vi "Measurement Logic.vi"(8 "error in":errorcluster, 11 "Measurement Configuration":T3={"Input Voltage in V"=4.0, "Nominal Output Voltage in V"=3.3, "Start"=0.03, "Stop"=0.43, "Step"=0.01, "Input SMU"="DPS_4145_1/1", "Load SMU"="DPS_4145_1/3", "Input DMM"="DMM1", "Load DMM"="DMM2"}) -> (0 "error out":errorcluster, 3 "Measurement Results":T2 {"Load Regulation (mV/mA)" format="%#.5g"})   [LabVIEW 2020, in "LoadRegulation.lvlib"]
uses:
  LoadRegulation.lvlib
  Measurement Configuration.ctl
  Measurement Results.ctl
  Reusables/TestResults.ctl
  Reusables/TestInputs.ctl
  Reusables/Advanced Settings.ctl
  Reusables/Prepare Fn Configurations.ctl
  Reusables/Load Output Function.ctl
  Reusables/Stimulus And Measure.ctl
  1892a527-43d9-4058-946b-211879b654a6.vi
panel:
  out "Load Regulation (mV/mA)":dbl format="%#.3g"
  out "Load Regulation (%)":dbl format="%#.3g"
  out "Test Results":T1
  out "Load Regulation":cluster{"Iload (mA)":dbl[], "Vout (V)":dbl[]}(graph)
  # "Below outputs could be used to debug or verify when we run this vi as standalone"
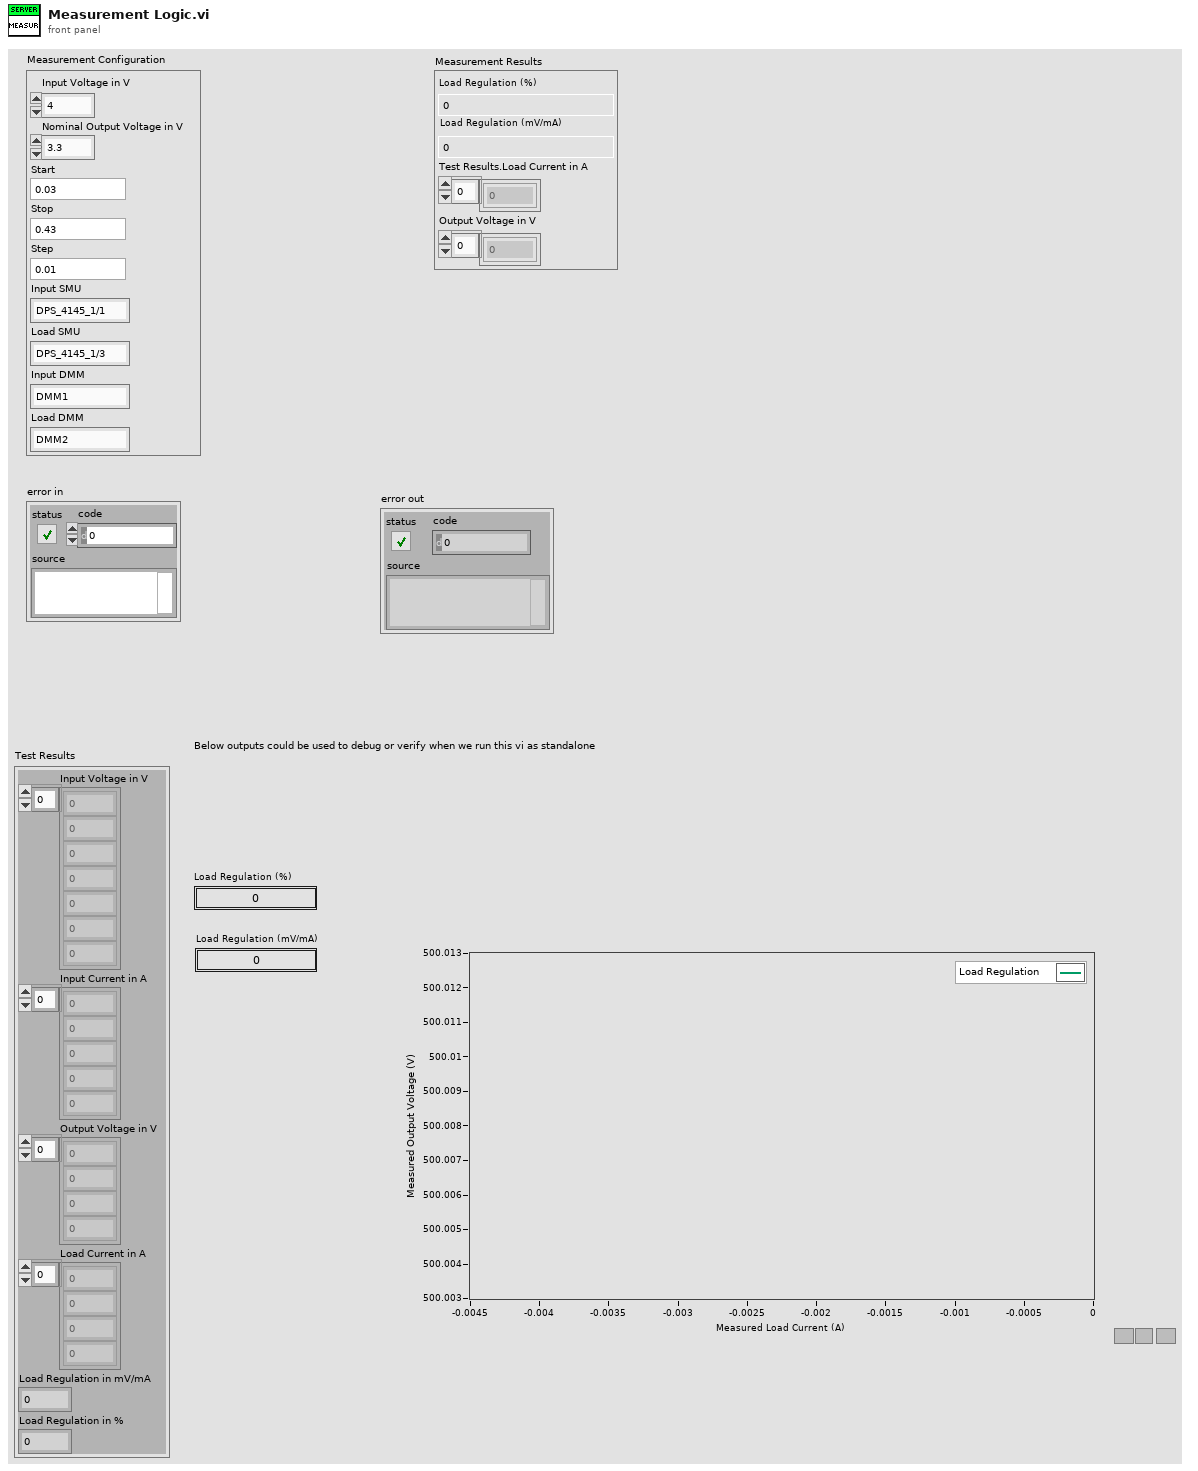
[diagram p1: front panel]
types:
  T1 = typedef "LoadRegulation.lvlib/TestResults.ctl" = cluster{"Input Voltage in V":dbl[], "Input Current in A":dbl[], "Output Voltage in V":dbl[], "Load Current in A":dbl[], "Load Regulation in mV/mA":dbl, "Load Regulation in %":dbl}
  T2 = typedef "LoadRegulation.lvlib/Measurement Results.ctl" = cluster{"Load Regulation (%)":dbl, "Load Regulation (mV/mA)":dbl, "Test Results.Load Current in A":dbl[], "Output Voltage in V":dbl[]}
  T3 = typedef "LoadRegulation.lvlib/Measurement Configuration.ctl" = cluster{"Input Voltage in V":dbl, "Nominal Output Voltage in V":dbl, "Start":dbl, "Stop":dbl, "Step":dbl, "Input SMU":string, "Load SMU":string, "Input DMM":string, "Load DMM":string}
  T4 = typedef "LoadRegulation.lvlib/TestInputs.ctl" = cluster{"Input Voltage in V":dbl, "Load Current in A":dbl[], "Nominal Output Voltage in V":dbl, "Advance Setting":T5}
  T5 = typedef "Advanced Settings.ctl" = cluster{"Prepare":T6, "Stimulus And Measure":T8}
  T6 = typedef "Prepare Fn Configurations.ctl" = cluster{"Load SMU Output Function":T7}
  T7 = typedef "Load Output Function.ctl" = enum16{"VoltageSource", "CurrentSource"}
  T8 = typedef "Stimulus And Measure.ctl" = cluster{"Loop Delay in milliSecond":u32}
  T9 = cluster{"Test Inputs":T4, "Test Results":T1, "Test Results[][]":string[][], "Input SMU":refnum<k15>, "Input DMM":refnum<k15>, "Load DMM":refnum<k15>, "Load SMU":refnum<k15>}
  T10 = cluster{"Load Current in A":dbl[], "Output Voltage in V":dbl[]}
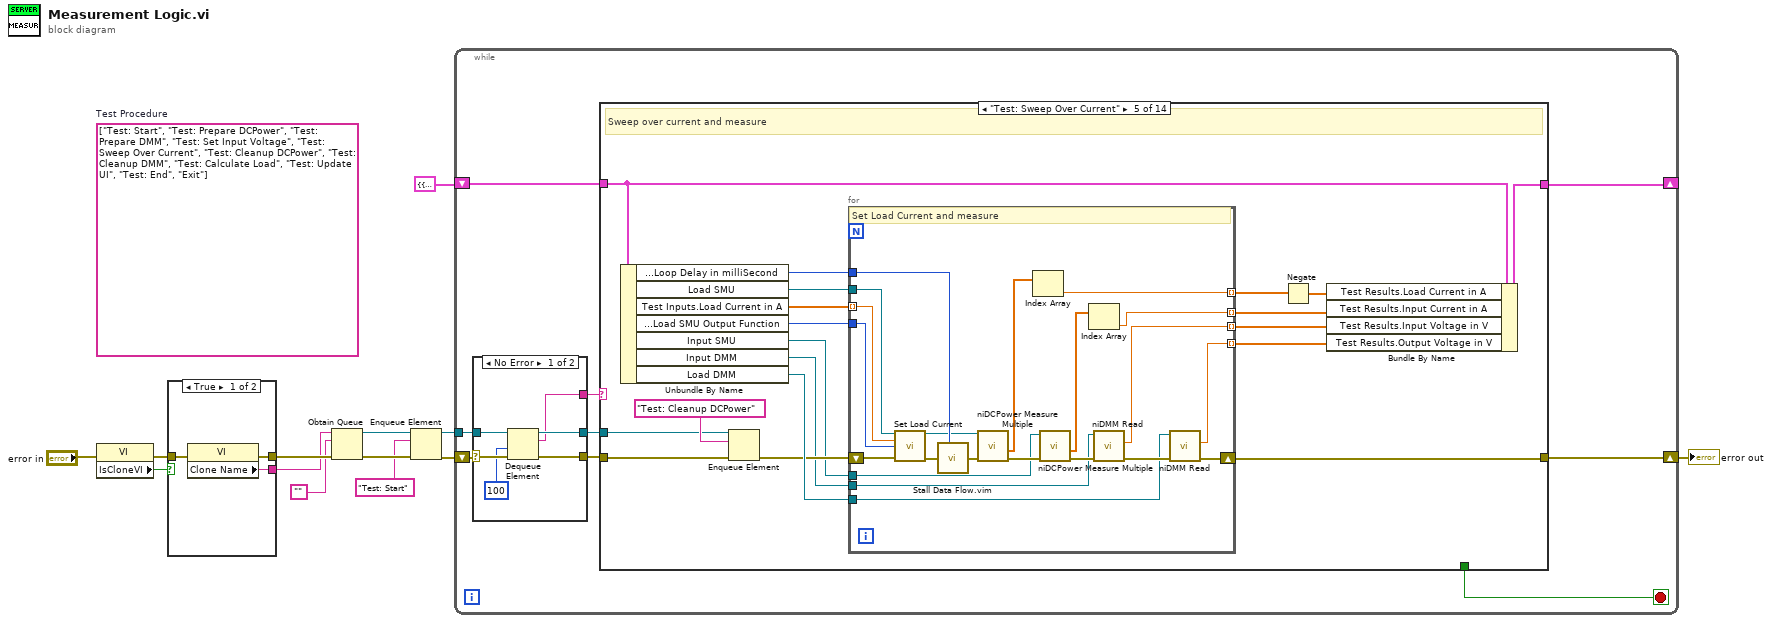
[diagram p0: block diagram]
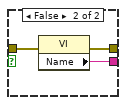
[diagram p2: hidden frame]
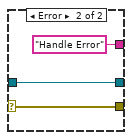
[diagram p3: hidden frame]
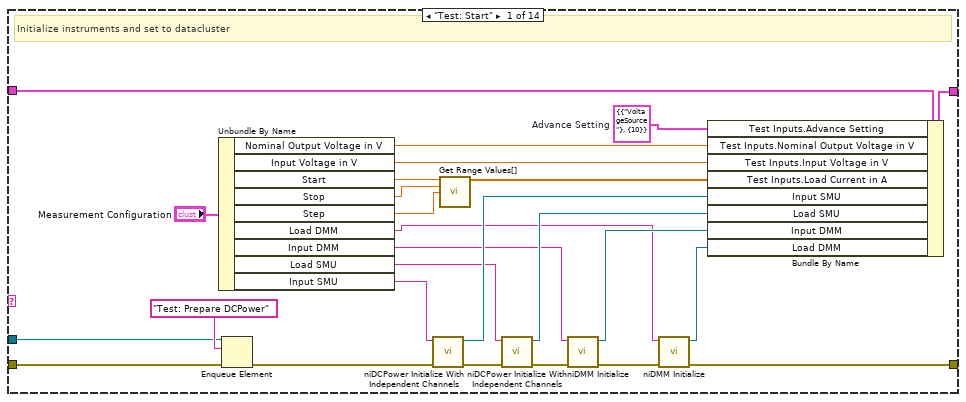
[diagram p4: hidden frame]
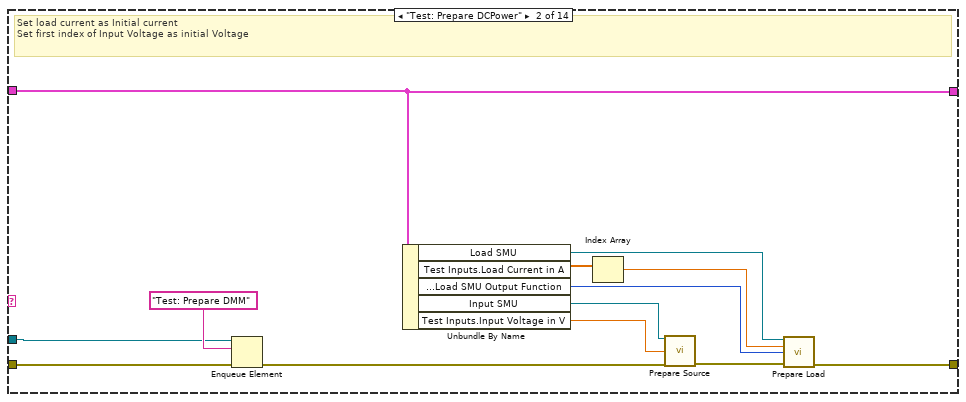
[diagram p5: hidden frame]
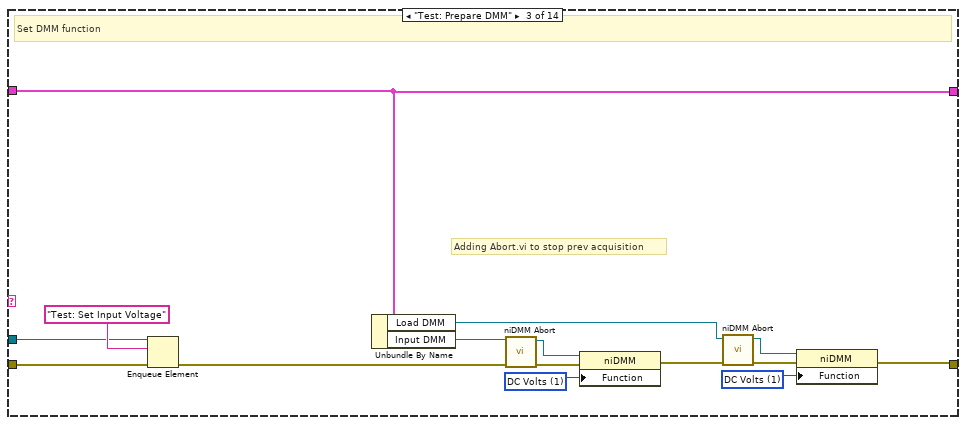
[diagram p6: hidden frame]
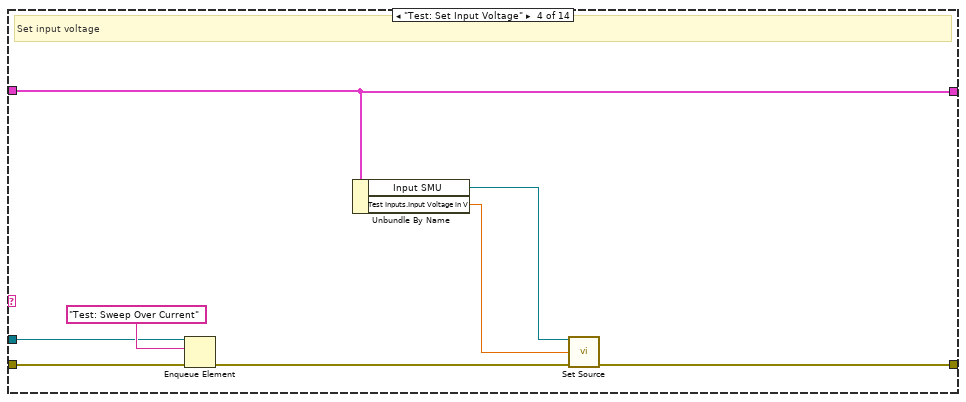
[diagram p7: hidden frame]
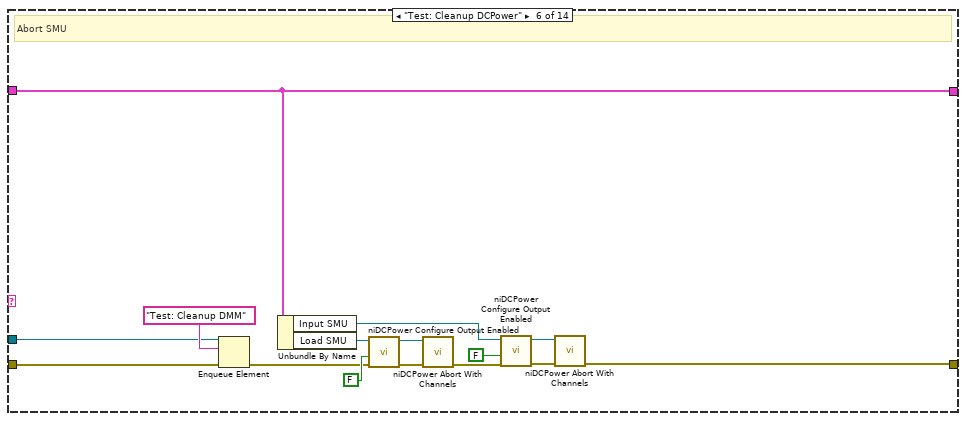
[diagram p8: hidden frame]
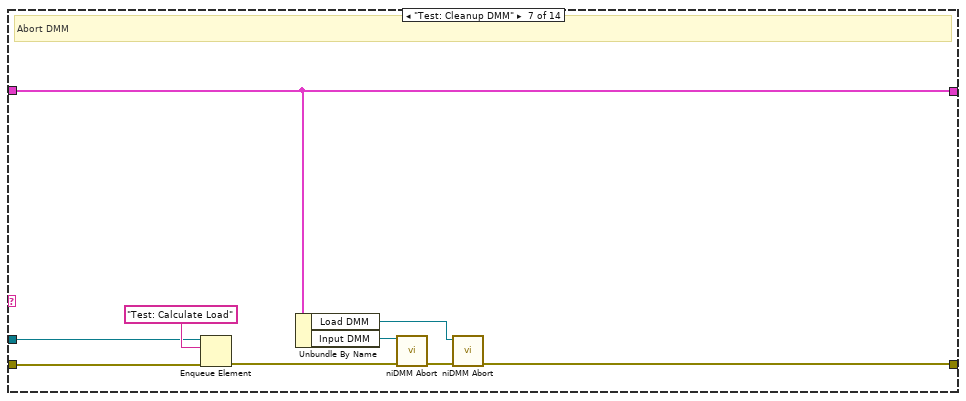
[diagram p9: hidden frame]
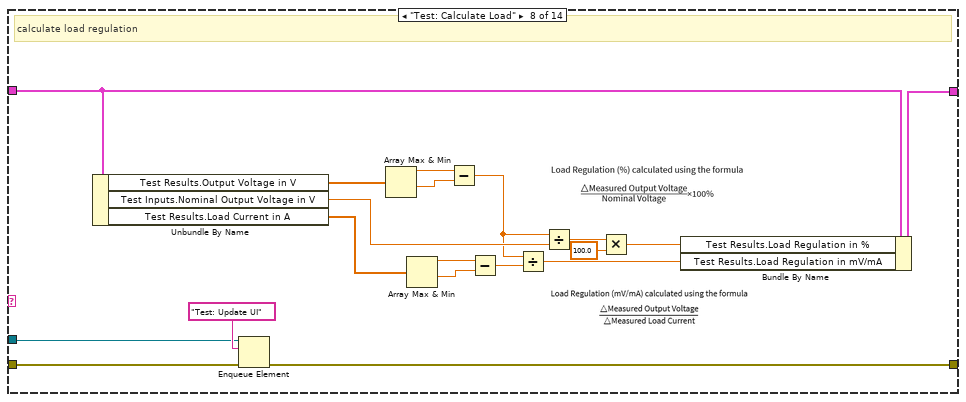
[diagram p10: hidden frame]
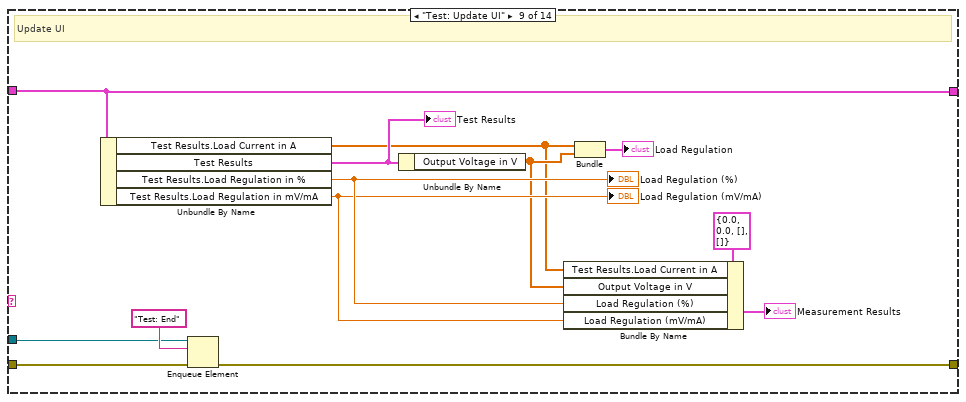
[diagram p11: hidden frame]
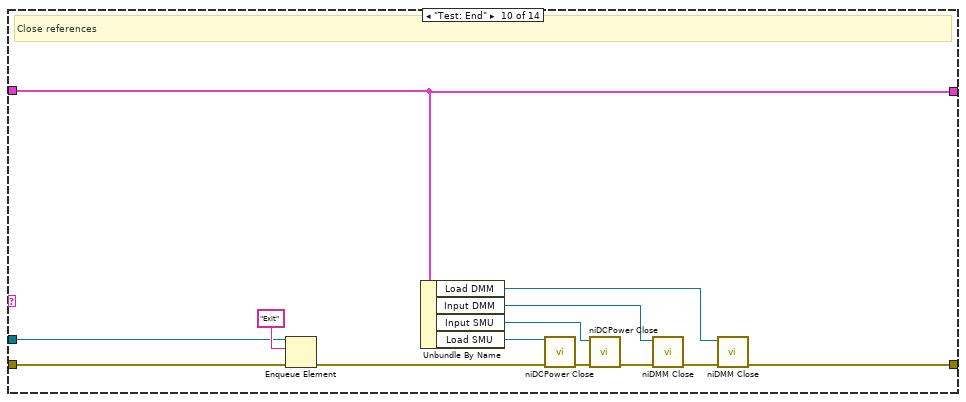
[diagram p12: hidden frame]
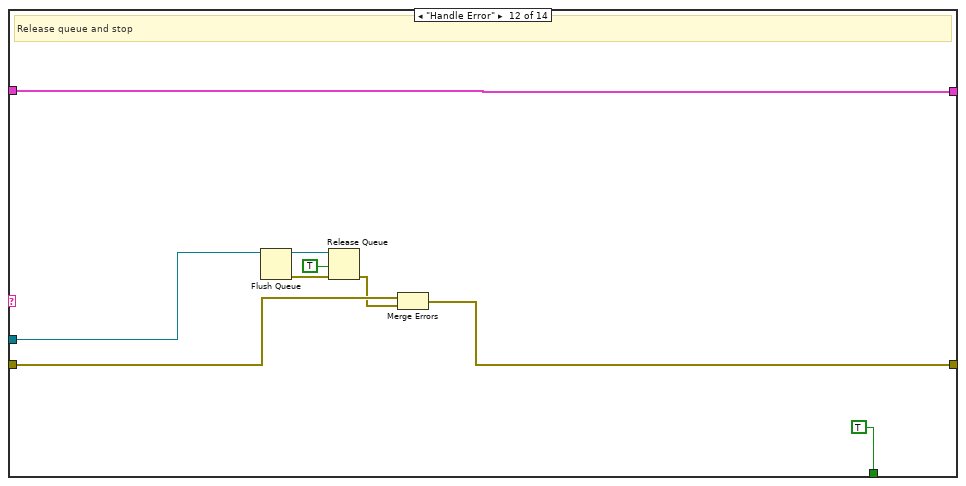
[diagram p14: hidden frame]
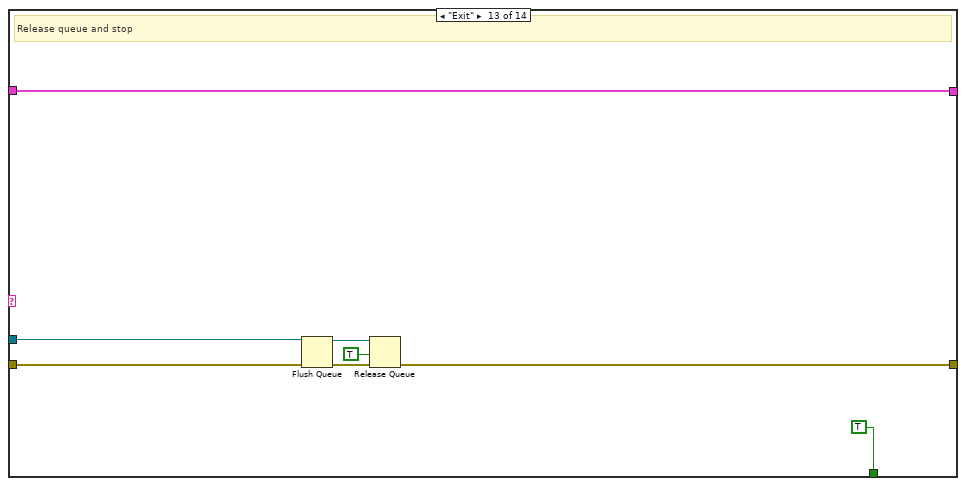
[diagram p15: hidden frame]
diagram:
  (unwired) string[] ["Test: Start", "Test: Prepare DCPower", "Test: Prepare DMM", "Test: Set Input Voltage", "Test: Sweep Over Current", "Test: Cleanup DCPower", "Test: Cleanup DMM", "Test: Calculate Load", "Test: Update UI", "Test: End", "Exit"]  # Test Procedure
  n1 = property class="VI"(error in="error in") -> (error out=w4:errorcluster, "IsCloneVI"=w5:bool)  [unwired: 1 in, 1 out]
  n2 = case shown="True" w5 {
    tunnel: [w16 w19] -> w11
    tunnel: [w15 w18] -> w10
    tunnel: w4 -> [w14 w17]
    frame True {
      n3 = property class="VI"(error in=w14) -> (error out=w16:errorcluster, "Clone Name"=w15:string)  [unwired: 1 in, 1 out]
    }
    frame False {
      n4 = property class="VI"(error in=w17) -> (error out=w19:errorcluster, "Name"=w18:string)  [unwired: 1 in, 1 out]
    }
  }
  n5 = Obtain Queue(name (unnamed)=w10, element data type="", error in (no error)=w11) -> (queue out=w8:refnum<queue>, error out=w9:errorcluster)  [unwired: 2 in, 1 out]
  n6 = Enqueue Element(queue=w8, element="Test: Start", error in (no error)=w9) -> (queue out=w2:refnum<queue>, error out=w1:errorcluster)  [unwired: 1 in, 1 out]
  n7 = while {
    tunnel: w2 -> [w23]
    shift-right: [w28] -> w12
    shift-left: w1 -> [w24]
    shift-right: [w26] -> _
    shift-left: T9 {"Test Inputs"={"Input Voltage in V"=0.0, "Load Current in A"=[], "Nominal Output Voltage in V"=0.0, "Advance Setting"={"Prepare"={"Load SMU Output Function"=enum."VoltageSource"}, "Stimulus And Measure"={"Loop Delay in milliSecond"=1}}}, "Test Results"={"Input Voltage in V"=[], "Input Current in A"=[], "Output Voltage in V"=[], "Load Current in A"=[], "Load Regulation in mV/mA"=0.0, "Load Regulation in %"=0.0}, "Test Results[][]"=[], "Input SMU"="", "Input DMM"="", "Load DMM"="", "Load SMU"=""} -> [w27]
    stop <- w25 stop-if-true
    n8 = case shown="No Error" w24 {
      selector: w24 -> [w34 w37]
      tunnel: [w33 w37] -> w20
      tunnel: w23 -> [w32 w36]
      tunnel: [w31 w36] -> w21
      tunnel: [w30 "Handle Error"] -> w22
      frame No Error {
        n9 = Dequeue Element(queue=w32, timeout in ms (-1)=100, error in (no error)=w34) -> (queue out=w31:refnum<queue>, element=w30:string, error out=w33:errorcluster)  [unwired: 1 out]
      }
      frame Error {
      }
    }
    n10 = case shown="\"Test: Sweep Over Current\"" w22 {
      tunnel: w21 -> [w43 w66 w79 w94 w106 w140 w155 w164 w183 w196 _ w211 w220 _]
      tunnel: w20 -> [w42 w67 w77 w92 w104 w142 w156 w165 w184 w197 w210 w217 w222 w228]
      tunnel: [w58 w70 w82 w96 w110 w151 w161 w166 w185 w202 w210 w218 w221 w228] -> w28
      tunnel: w27 -> [w62 w75 w88 w99 w108 w150 w163 w168 w193 w208 w209 w219 w227 w229]
      tunnel: [w63 w75 w88 w99 w109 w150 w163 w169 w193 w208 w209 w219 w227 w229] -> w26
      tunnel: [_ _ _ _ _ _ _ _ _ _ _ TRUE TRUE _] -> w25
      frame "Test: Start" {
        w40 = T5 {"Prepare"={"Load SMU Output Function"=enum."VoltageSource"}, "Stimulus And Measure"={"Loop Delay in milliSecond"=10}}  # Advance Setting
        # "Initialize instruments and set to datacluster"
        n11 = Unbundle By Name("Measurement Configuration") -> ("Nominal Output Voltage in V"=w53:dbl, "Input Voltage in V"=w38:dbl, "Start"=w51:dbl, "Stop"=w50:dbl, "Step"=w49:dbl, "Load DMM"=w45:string, "Input DMM"=w46:string, "Load SMU"=w47:string, "Input SMU"=w48:string)
        n12 = Enqueue Element(queue=w43, element="Test: Prepare DCPower", error in (no error)=w42) -> (error out=w41:errorcluster)  [unwired: 1 in, 2 out]
        n13 = call <instrlib>:"niDCPower Initialize With Independent Channels.vi"("error in (no error)"=w41, "resource name"=w48) -> ("error out"=w57:errorcluster, "instrument handle out"=w61:refnum<k15>)  [unwired: 8 in]
        n14 = call "Get Range Values[].vi"("Start"=w51, "Stop"=w50, "Step Size"=w49) -> ("Values[]"=w39:dbl[])  [unwired: 12 in]
        n15 = call <instrlib>:"niDCPower Initialize With Independent Channels.vi"("error in (no error)"=w57, "resource name"=w47) -> ("error out"=w56:errorcluster, "instrument handle out"=w54:refnum<k15>)  [unwired: 8 in]
        n16 = call <instrlib>:"niDMM Initialize.vi"("error in (no error)"=w56, "Instrument Descriptor"=w46) -> ("error out"=w59:errorcluster, "instrument handle out"=w55:refnum<k15>)  [unwired: 8 in]
        n17 = call <instrlib>:"niDMM Initialize.vi"("error in (no error)"=w59, "Instrument Descriptor"=w45) -> ("error out"=w58:errorcluster, "instrument handle out"=w60:refnum<k15>)  [unwired: 8 in]
        n18 = Bundle By Name(cluster=w62, "Test Inputs.Advance Setting"=w40, "Test Inputs.Nominal Output Voltage in V"=w53, "Test Inputs.Input Voltage in V"=w38, "Test Inputs.Load Current in A"=w39, "Input SMU"=w61, "Load SMU"=w54, "Input DMM"=w55, "Load DMM"=w60) -> (w63:T9)
      }
      frame "Test: Prepare DCPower" {
        # "Set load current as Initial current\nSet first index of Input Voltage as initial Voltage"
        n19 = Enqueue Element(queue=w66, element="Test: Prepare DMM", error in (no error)=w67) -> (error out=w68:errorcluster)  [unwired: 1 in, 2 out]
        n20 = Unbundle By Name(w75) -> ("Load SMU"=w73:refnum<k15>, "Test Inputs.Load Current in A"=w72:dbl[], "Test Inputs.Advance Setting.Prepare.Load SMU Output Function"=w64:T7, "Input SMU"=w74:refnum<k15>, "Test Inputs.Input Voltage in V"=w76:dbl)
        n21 = Index Array(array=w72) -> (element=w65:dbl)  [unwired: 1 in]
        n22 = call "Prepare Source.vi"("instrument handle"=w74, "Initial Voltage Level (V)"=w76, "error in (no error)"=w68) -> ("error out"=w71:errorcluster)  [unwired: 12 in]
        n23 = call "Prepare Load.vi"("instrument handle"=w73, "Load Current Level (A)"=w65, "Load Output Function"=w64, "error in (no error)"=w71) -> ("error out"=w70:errorcluster)  [unwired: 11 in]
      }
      frame "Test: Prepare DMM" {
        w84 = 1 items=["DC Volts"=1, "AC Volts"=2, "DC Current"=3, "AC Current"=4, "2-Wire Resistance"=5, "4-Wire Resistance"=101, "Frequency"=104, "Period"=105, "AC Volts DC Coupled"=1001, "Diode"=1002, "Waveform Voltage"=1003, "Waveform Current"=1004, "Capacitance"=1005, "Inductance"=1006, "Temperature"=108] ("Configuration:Function")
        w91 = 1 items=["DC Volts"=1, "AC Volts"=2, "DC Current"=3, "AC Current"=4, "2-Wire Resistance"=5, "4-Wire Resistance"=101, "Frequency"=104, "Period"=105, "AC Volts DC Coupled"=1001, "Diode"=1002, "Waveform Voltage"=1003, "Waveform Current"=1004, "Capacitance"=1005, "Inductance"=1006, "Temperature"=108] ("Configuration:Function")
        # "Adding Abort.vi to stop prev acquisition"
        # "Set DMM function"
        n24 = Enqueue Element(queue=w79, element="Test: Set Input Voltage", error in (no error)=w77) -> (error out=w78:errorcluster)  [unwired: 1 in, 2 out]
        n25 = Unbundle By Name(w88) -> ("Load DMM"=w81:refnum<k15>, "Input DMM"=w87:refnum<k15>)
        n26 = call <instrlib>:"niDMM Abort.vi"("error in (no error)"=w78, "instrument handle"=w87) -> ("error out"=w90:errorcluster, "instrument handle out"=w89:refnum<k15>)  [unwired: 8 in]
        n27 = property class="niDMM"(reference=w89, error in=w90, "Function"=w91) -> (error out=w83:errorcluster)  [unwired: 1 out]
        n28 = call <instrlib>:"niDMM Abort.vi"("error in (no error)"=w83, "instrument handle"=w81) -> ("error out"=w85:errorcluster, "instrument handle out"=w86:refnum<k15>)  [unwired: 8 in]
        n29 = property class="niDMM"(reference=w86, error in=w85, "Function"=w84) -> (error out=w82:errorcluster)  [unwired: 1 out]
      }
      frame "Test: Set Input Voltage" {
        # "Set input voltage"
        n30 = Enqueue Element(queue=w94, element="Test: Sweep Over Current", error in (no error)=w92) -> (error out=w93:errorcluster)  [unwired: 1 in, 2 out]
        n31 = Unbundle By Name(w99) -> ("Input SMU"=w98:refnum<k15>, "Test Inputs.Input Voltage in V"=w97:dbl)
        n32 = call "Set Source.vi"("instrument handle in"=w98, "Vin in V"=w97, "error in (no error)"=w93) -> ("error out"=w96:errorcluster)  [unwired: 11 in, 1 out]
      }
      frame "Test: Sweep Over Current" {
        # "Sweep over current and measure"
        n33 = Unbundle By Name(w108) -> ("Test Inputs.Advance Setting.Stimulus And Measure.Loop Delay in milliSecond"=w116:u32, "Load SMU"=w118:refnum<k15>, "Test Inputs.Load Current in A"=w117:dbl[], "Test Inputs.Advance Setting.Prepare.Load SMU Output Function"=w103:T7, "Input SMU"=w100:refnum<k15>, "Input DMM"=w101:refnum<k15>, "Load DMM"=w115:refnum<k15>)
        n34 = Enqueue Element(queue=w106, element="Test: Cleanup DCPower", error in (no error)=w104) -> (error out=w105:errorcluster)  [unwired: 1 in, 2 out]
        n35 = for {
          tunnel: w118 -> [w138]
          tunnel: w117 -> [w121] mode=indexing
          tunnel: w116 -> [w136]
          tunnel: w101 -> [w129]
          tunnel: w115 -> [w128]
          tunnel: [w122] -> w114 mode=indexing
          tunnel: [w123] -> w113 mode=indexing
          tunnel: [w127] -> w112 mode=indexing
          tunnel: [w126] -> w111 mode=indexing
          shift-right: [w125] -> w110
          shift-left: w105 -> [w139]
          tunnel: w103 -> [w120]
          tunnel: w100 -> [w119]
          # "Set Load Current and measure"
          n36 = call "Set Load Current.vi"("instrument handle in"=w138, "current level"=w121, "OutputFunction"=w120, "error in (no error)"=w139) -> ("instrument handle out"=w124:refnum<k15>, "error out"=w137:errorcluster)  [unwired: 10 in]
          n37 = call "Stall Data Flow.vim"("value in"=w137, "milliseconds to wait"=w136) -> ("value out"=w130:errorcluster)  [unwired: 1 out]
          n38 = call <instrlib>:"niDCPower Measure Multiple.vi"("error in (no error)"=w130, "instrument handle"=w124) -> ("error out"=w132:errorcluster, "current measurements"=w135:dbl[])  [unwired: 6 in, 2 out]
          n39 = Index Array(array=w135) -> (element=w123:dbl)  [unwired: 1 in]
          n40 = call <instrlib>:"niDCPower Measure Multiple.vi"("error in (no error)"=w132, "instrument handle"=w119) -> ("error out"=w131:errorcluster, "current measurements"=w133:dbl[])  [unwired: 6 in, 2 out]
          n41 = Index Array(array=w133) -> (element=w122:dbl)  [unwired: 1 in]
          n42 = call <instrlib>:"niDMM Read.vi"("error in (no error)"=w131, "instrument handle"=w129) -> ("error out"=w134:errorcluster, "Measurement"=w127:dbl)  [unwired: 7 in, 1 out]
          n43 = call <instrlib>:"niDMM Read.vi"("error in (no error)"=w134, "instrument handle"=w128) -> ("error out"=w125:errorcluster, "Measurement"=w126:dbl)  [unwired: 7 in, 1 out]
        }
        n44 = Negate(x=w113) -> (-x=w102:dbl[])
        n45 = Bundle By Name(cluster=w108, "Test Results.Load Current in A"=w102, "Test Results.Input Current in A"=w114, "Test Results.Input Voltage in V"=w112, "Test Results.Output Voltage in V"=w111) -> (w109:T9)
      }
      frame "Test: Cleanup DCPower" {
        # "Abort SMU"
        n46 = Enqueue Element(queue=w140, element="Test: Cleanup DMM", error in (no error)=w142) -> (error out=w141:errorcluster)  [unwired: 1 in, 2 out]
        n47 = Unbundle By Name(w150) -> ("Input SMU"=w149:refnum<k15>, "Load SMU"=w144:refnum<k15>)
        n48 = call <instrlib>:"niDCPower Configure Output Enabled.vi"("error in (no error)"=w141, "output enabled"=FALSE, "instrument handle"=w144) -> ("error out"=w145:errorcluster, "instrument handle out"=w148:refnum<k15>)  [unwired: 7 in]
        n49 = call <instrlib>:"niDCPower Abort With Channels.vi"("error in (no error)"=w145, "instrument handle"=w148) -> ("error out"=w146:errorcluster)  [unwired: 8 in, 1 out]
        n50 = call <instrlib>:"niDCPower Configure Output Enabled.vi"("error in (no error)"=w146, "output enabled"=FALSE, "instrument handle"=w149) -> ("error out"=w153:errorcluster, "instrument handle out"=w152:refnum<k15>)  [unwired: 7 in]
        n51 = call <instrlib>:"niDCPower Abort With Channels.vi"("error in (no error)"=w153, "instrument handle"=w152) -> ("error out"=w151:errorcluster)  [unwired: 8 in, 1 out]
      }
      frame "Test: Cleanup DMM" {
        # "Abort DMM"
        n52 = Enqueue Element(queue=w155, element="Test: Calculate Load", error in (no error)=w156) -> (error out=w157:errorcluster)  [unwired: 1 in, 2 out]
        n53 = Unbundle By Name(w163) -> ("Load DMM"=w160:refnum<k15>, "Input DMM"=w159:refnum<k15>)
        n54 = call <instrlib>:"niDMM Abort.vi"("error in (no error)"=w157, "instrument handle"=w159) -> ("error out"=w162:errorcluster)  [unwired: 8 in, 1 out]
        n55 = call <instrlib>:"niDMM Abort.vi"("error in (no error)"=w162, "instrument handle"=w160) -> ("error out"=w161:errorcluster)  [unwired: 8 in, 1 out]
      }
      frame "Test: Calculate Load" {
        # "calculate load regulation"
        n56 = Unbundle By Name(w168) -> ("Test Results.Output Voltage in V"=w179:dbl[], "Test Inputs.Nominal Output Voltage in V"=w177:dbl, "Test Results.Load Current in A"=w174:dbl[])
        n57 = Enqueue Element(queue=w164, element="Test: Update UI", error in (no error)=w165) -> (error out=w166:errorcluster)  [unwired: 1 in, 2 out]
        n58 = Array Max & Min(array=w179) -> (max value=w182:dbl, min value=w178:dbl)  [unwired: 2 out]
        n59 = Array Max & Min(array=w174) -> (max value=w175:dbl, min value=w176:dbl)  [unwired: 2 out]
        n60 = Subtract(x=w182, y=w178) -> (x-y=w173:dbl)
        n61 = Subtract(x=w175, y=w176) -> (x-y=w172:dbl)
        n62 = Divide(x=w173, y=w172) -> (x/y=w171:dbl)
        n63 = Divide(x=w173, y=w177) -> (x/y=w181:dbl)
        n64 = Multiply(x=w181, y=100.0) -> (x*y=w180:dbl)
        n65 = Bundle By Name(cluster=w168, "Test Results.Load Regulation in %"=w180, "Test Results.Load Regulation in mV/mA"=w171) -> (w169:T9)
      }
      frame "Test: Update UI" {
        # "Update UI"
        n66 = Unbundle By Name(w193) -> ("Test Results.Load Current in A"=w187:dbl[], "Test Results"=w195:T1, "Test Results.Load Regulation in %"=w190:dbl, "Test Results.Load Regulation in mV/mA"=w189:dbl)
        "Test Results" <- w195
        "Load Regulation (%)" <- w190
        "Load Regulation (mV/mA)" <- w189
        n67 = Enqueue Element(queue=w183, element="Test: End", error in (no error)=w184) -> (error out=w185:errorcluster)  [unwired: 1 in, 2 out]
        n68 = Unbundle By Name(w195) -> ("Output Voltage in V"=w188:dbl[])
        n69 = Bundle By Name(cluster=T2 {"Load Regulation (%)"=0.0, "Load Regulation (mV/mA)"=0.0, "Test Results.Load Current in A"=[], "Output Voltage in V"=[]} ("Measurement Results"), "Test Results.Load Current in A"=w187, "Output Voltage in V"=w188, "Load Regulation (%)"=w190, "Load Regulation (mV/mA)"=w189) -> (→"Measurement Results":T2)
        n70 = Bundle("Load Current in A"=w187, "Output Voltage in V"=w188) -> (→"Load Regulation":T10)  [unwired: 1 in]
      }
      frame "Test: End" {
        # "Close references"
        n71 = Enqueue Element(queue=w196, element="Exit", error in (no error)=w197) -> (error out=w198:errorcluster)  [unwired: 1 in, 2 out]
        n72 = Unbundle By Name(w208) -> ("Load DMM"=w203:refnum<k15>, "Input DMM"=w204:refnum<k15>, "Input SMU"=w207:refnum<k15>, "Load SMU"=w201:refnum<k15>)
        n73 = call <instrlib>:"niDCPower Close.vi"("error in (no error)"=w198, "instrument handle"=w201) -> ("error out"=w200:errorcluster)  [unwired: 9 in]
        n74 = call <instrlib>:"niDCPower Close.vi"("error in (no error)"=w200, "instrument handle"=w207) -> ("error out"=w206:errorcluster)  [unwired: 9 in]
        n75 = call <instrlib>:"niDMM Close.vi"("error in (no error)"=w206, "instrument handle"=w204) -> ("error out"=w205:errorcluster)  [unwired: 9 in]
        n76 = call <instrlib>:"niDMM Close.vi"("error in (no error)"=w205, "instrument handle"=w203) -> ("error out"=w202:errorcluster)  [unwired: 9 in]
      }
      frame "----Misc------" {
      }
      frame "Handle Error" {
        # "Release queue and stop"
        n77 = Flush Queue(queue=w211) -> (queue out=w215:refnum<queue>, error out=w214:errorcluster)  [unwired: 1 in, 1 out]
        n78 = Release Queue(queue=w215, force destroy? (F)=TRUE, error in (no error)=w214) -> (error out=w212:errorcluster)  [unwired: 2 out]
        n79 = Merge Errors(w217, w212) -> (w218:errorcluster)
      }
      frame "Exit" {
        # "Release queue and stop"
        n80 = Flush Queue(queue=w220, error in (no error)=w222) -> (queue out=w225:refnum<queue>, error out=w224:errorcluster)  [unwired: 1 out]
        n81 = Release Queue(queue=w225, force destroy? (F)=TRUE, error in (no error)=w224) -> (error out=w221:errorcluster)  [unwired: 2 out]
      }
      frame "", Default {
        # "Do nothing"
      }
    }
  }
  "error out" <- w12
